vi "WriteLogFile.vi"(6 "Prepend TimeStamp":bool=TRUE, 8 "error in (no error)":errorcluster, 9 "Log Message":string, 11 "LogFile":path) -> (0 "error out":errorcluster)   [LabVIEW 2025]
doc: "Use this template to build a VI to use as a subVI."
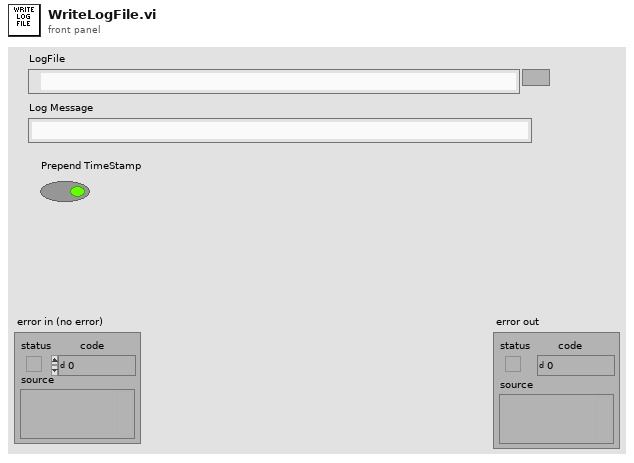
[diagram p1: front panel]
types:
  T1 = enum16{"open", "replace", "create", "open or create", "replace or create", "replace or create with confirmation"}
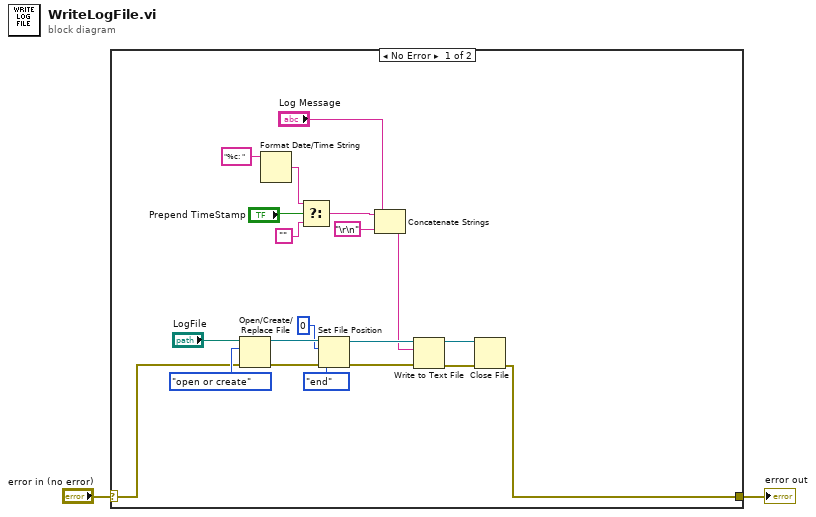
[diagram p0: block diagram]
diagram:
  n1 = case shown="No Error" "error in (no error)" {
    selector: "error in (no error)" -> [w20 w23]
    tunnel: [w11 w23] -> w1
    frame No Error {
      n2 = Open/Create/Replace File(file path (use dialog)="LogFile", error in=w20, operation (0:open)=T1."open or create") -> (refnum out=w18:refnum<file>, error out=w19:errorcluster)  [unwired: 3 in, 1 out]
      n3 = Format Date/Time String(time format string (%c)="%c: ") -> (date/time string=w8:string)  [unwired: 2 in]
      n4 = Select(t=w8, s="Prepend TimeStamp", f="") -> (s? t:f=w4:string)
      n5 = Set File Position(offset (in bytes) (0)=i64 0, refnum=w18, from (0:start)=enum16{"start", "end", "current"}."end", error in=w19) -> (refnum out=w14:refnum<file>, error out=w15:errorcluster)
      n6 = Concatenate Strings(w4, "Log Message", "\r\n") -> (w5:string)
      n7 = Write to Text File(file (use dialog)=w14, text=w5, error in=w15) -> (refnum out=w12:refnum<file>, error out=w13:errorcluster)  [unwired: 1 in, 1 out]
      n8 = Close File(refnum=w12, error in=w13) -> (error out=w11:errorcluster)  [unwired: 1 out]
    }
    frame Error {
    }
  }
  "error out" <- w1
